vi "Close.vi"(8 "error in (no error)":errorcluster, 11 "LabVIEW Build Script in":refnum<class "LabVIEW Build Script.lvclass">) -> (0 "error out":errorcluster, 3 "LabVIEW Build Script out":refnum<class "LabVIEW Build Script.lvclass">)   [LabVIEW 2021, in "LabVIEW Build Script.lvclass"]
uses:
  LabVIEW Build Script.lvclass
  LabVIEW Build Script.lvclass/LabVIEW Build Script.ctl
  Build Script Common/Build Script Common.lvlib
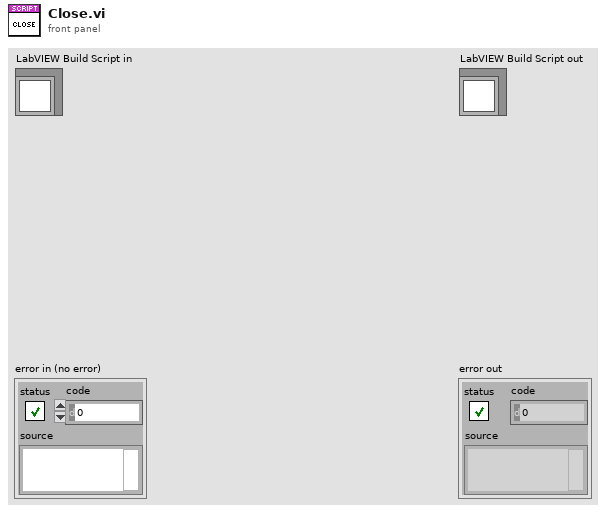
[diagram p1: front panel]
types:
  T1 = typedef "Build Script Common.lvlib/References.ctl" = cluster{"UI Display":refnum<vi>, "UI Display Valid":bool, "UI Semaphore":T2}
  T2 = typedef "Semaphore RefNum" = refnum<k1>
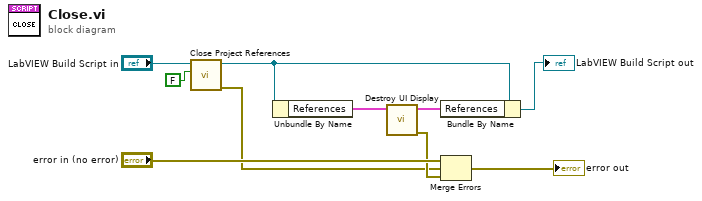
[diagram p0: block diagram]
diagram:
  n1 = call "Close Project References.vi"("Save All"=FALSE, "LabVIEW Build Script in"="LabVIEW Build Script in") -> ("error out"=w2:errorcluster, "LabVIEW Build Script out"=w7:refnum<class "LabVIEW Build Script.lvclass">)  [unwired: 8 in]
  n2 = Unbundle By Name(w7) -> ("References"=w8:T1)
  n3 = call "Destroy UI Display.vi"("References in"=w8) -> ("error out"=w3:errorcluster, "References out"=w6:T1)  [unwired: 9 in]
  n4 = Bundle By Name(cluster=w7, "References"=w6) -> (→"LabVIEW Build Script out":refnum<class "LabVIEW Build Script.lvclass">)
  n5 = Merge Errors("error in (no error)", w2, w3) -> (→"error out":errorcluster)
